vi "Auto Setup.vi"(8 "error in (no error)":errorcluster) -> ()   [LabVIEW 2019]
uses:
  <vilib>/Rock Robotics/Network Tables/NT Read String Array.vi
  <vilib>/Rock Robotics/Network Tables/NT Write Variant.vi
  2020 Robot/Framework/Robot Global Data.vi
  <vilib>/Rock Robotics/Network Tables/NT Write String Array.vi
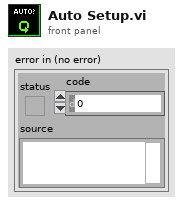
[diagram p1: front panel]
types:
  T1 = cluster{"Segment Name":string, "Type":enum16{"Accel Straight", "Const Straight", "Blend", "Circle"}, "Traj Pos Points":cluster{"x":dbl, "y":dbl, "th":dbl}[], "Traj Vel Points":cluster{"V":dbl, "th":dbl}[], "Accel Index":i32, "Decel Index":i32}[]
  T2 = cluster{"Trajectory Data":cluster{"Segment Name":string, "Type":enum16{"Accel Straight", "Const Straight", "Blend", "Circle"}, "Traj Pos Points":cluster{"x":dbl, "y":dbl, "th":dbl}[], "Traj Vel Points":cluster{"V":dbl, "th":dbl}[], "Accel Index":i32, "Decel Index":i32}[], "Points":cluster{"x":dbl, "y":dbl, "th":dbl}[]}
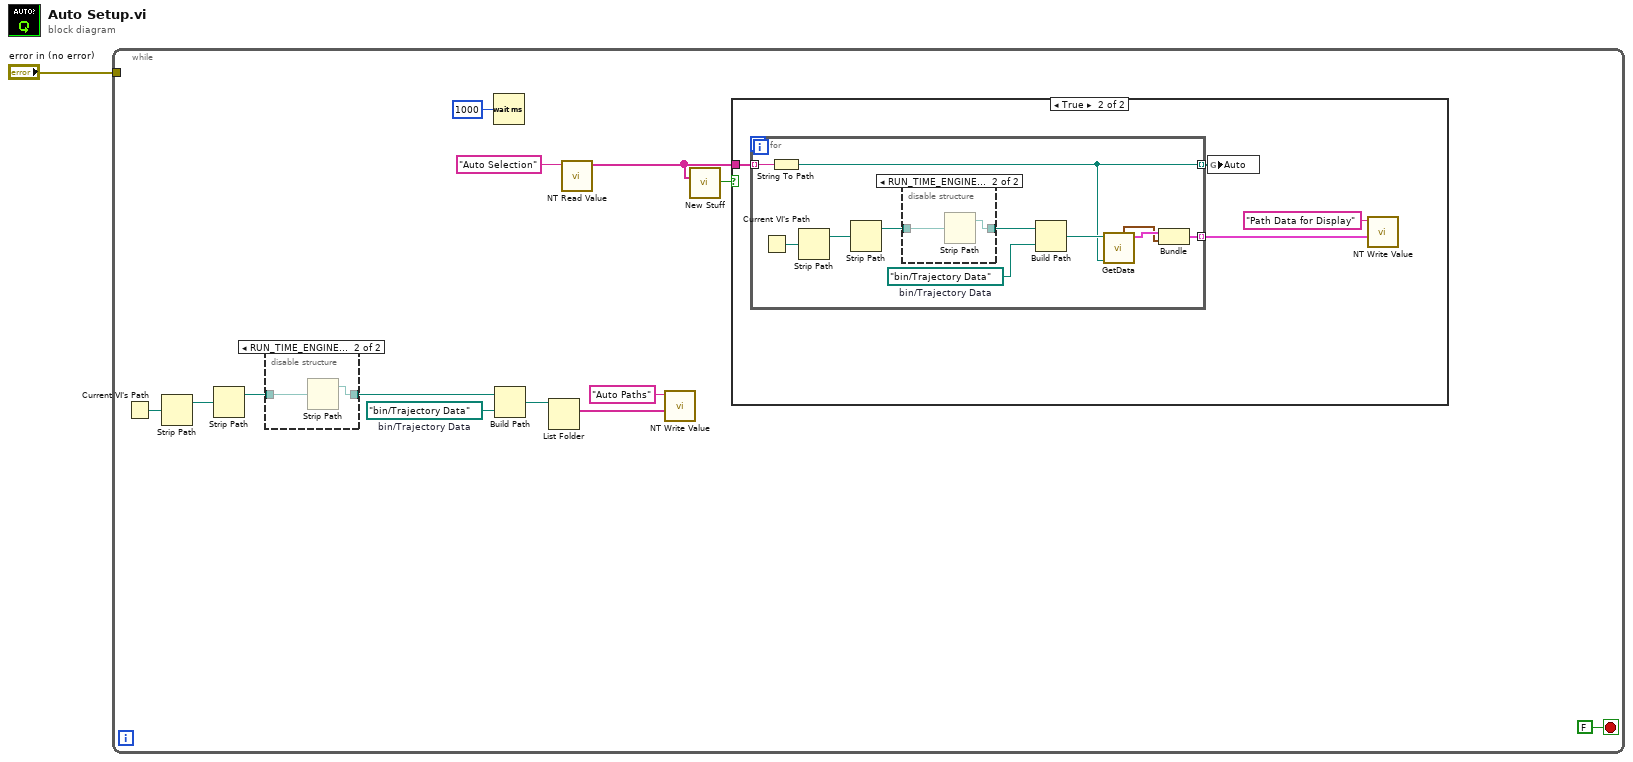
[diagram p0: block diagram]
diagram:
  n1 = while {
    tunnel: "error in (no error)" -> [_]
    stop <- FALSE stop-if-true
    w4 = path "bin/Trajectory Data"  # bin/Trajectory Data
    n2 = Current VI's Path() -> (path=w5:path)
    n3 = Strip Path(path=w5) -> (stripped path=w6:path)  [unwired: 1 out]
    n4 = Strip Path(path=w6) -> (stripped path=w8:path)  [unwired: 1 out]
    n5 = disable-structure shown="RUN_TIME_ENGINE==True, Default" {
      disable-tunnel: [w33 w34] -> w7
      disable-tunnel: w8 -> [w33 w35]
      frame condition #0 (active) {
      }
      frame condition #1 {
        n6 = Strip Path(path=w35) -> (stripped path=w34:path)  [unwired: 1 out]
      }
    }
    n7 = Wait (ms)(milliseconds to wait=u32 1000) -> ()  [unwired: 1 out]
    n8 = Build Path(base path=w7, name or relative path=w4) -> (appended path=w9:path)
    n9 = List Folder(path=w9) -> (filenames=w2:string[])  [unwired: 3 in, 3 out]
    n10 = call-poly <vilib>:"NT Read Value.vi"("Name"="Auto Selection") -> ("String Array"=w11:string[])  [unwired: 9 in, 1 out]
    n11 = call-poly <vilib>:"NT Write Value.vi"("String Array"=w2, "Name"="Auto Paths") -> ()  [unwired: 9 in, 1 out]
    n12 = call "New Stuff.vi"("Variant 4"=w11) -> ("x != y?"=w12:bool)  [unwired: 26 in]
    n13 = case shown="True" w12 {
      tunnel: w11 -> [_ w18]
      frame False {
      }
      frame True {
        n14 = for {
          tunnel: w18 -> [w29] mode=indexing
          tunnel: [w23] -> w17 mode=indexing
          tunnel: [w19] -> w15 mode=indexing
          w22 = path "bin/Trajectory Data"  # bin/Trajectory Data
          n15 = Current VI's Path() -> (path=w25:path)
          n16 = String To Path(string=w29) -> (path=w23:path)
          n17 = Strip Path(path=w25) -> (stripped path=w26:path)  [unwired: 1 out]
          n18 = Strip Path(path=w26) -> (stripped path=w28:path)  [unwired: 1 out]
          n19 = disable-structure shown="RUN_TIME_ENGINE==True, Default" {
            disable-tunnel: [w30 w31] -> w27
            disable-tunnel: w28 -> [w30 w32]
            frame condition #0 (active) {
            }
            frame condition #1 {
              n20 = Strip Path(path=w32) -> (stripped path=w31:path)  [unwired: 1 out]
            }
          }
          n21 = Build Path(base path=w27, name or relative path=w22) -> (appended path=w24:path)
          n22 = call "GetData.vi"("File"=w23, "file (use dialog)"=w24) -> ("Trajectory Data"=w21:T1, "Points"=w20:cluster{"x":dbl, "y":dbl, "th":dbl}[])  [unwired: 2 in, 6 out]
          n23 = Bundle("Trajectory Data"=w21, "Points"=w20) -> (w19:T2)  [unwired: 1 in]
        }
        n24 = global write "Robot Global Data.vi" "Auto"(w17) -> ()
        n25 = call-poly <vilib>:"NT Write Value.vi"("Variant"=w15, "Name"="Path Data for Display") -> ()  [unwired: 9 in, 1 out]
      }
    }
  }
